vi "clearWaveforms.vi"(8 "ErrorIn":errorcluster, 11 "AccelerationDataIn":waveform(dbl)[](array[waveform])) -> (0 "ErrorOut":errorcluster, 3 "AccelerationDataOut":waveform(dbl)[](array[waveform]))   [LabVIEW 2019]
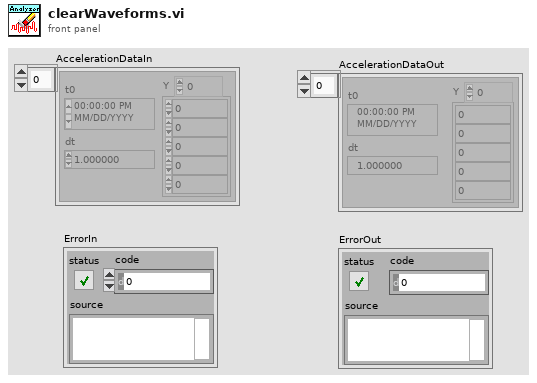
[diagram p1: front panel]
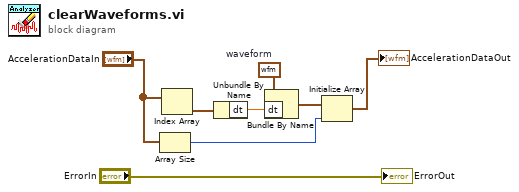
[diagram p0: block diagram]
diagram:
  w1 = waveform(dbl) {"t0"=timestamp(0 s since 1904-01-01), "dt"=0.0, "Y"=[]}  # waveform
  n1 = Array Size(array="AccelerationDataIn") -> (size(s)=w4:i32)
  n2 = Index Array(array="AccelerationDataIn") -> (element=w8:waveform(dbl))  [unwired: 1 in]
  n3 = Unbundle By Name(w8) -> ("dt"=w6:dbl)
  n4 = Bundle By Name(cluster=w1, "dt"=w6) -> (w5:waveform(dbl))
  n5 = Initialize Array(w5, w4) -> (→"AccelerationDataOut":waveform(dbl)[])
  "ErrorOut" <- "ErrorIn"
